vi "Node - Get Imported Ch Data.vi"(8 "error in (no error)":errorcluster) -> (0 "error out":errorcluster)   [LabVIEW 2016]
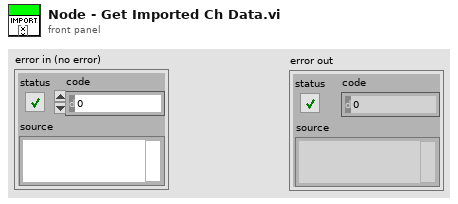
[diagram p1: front panel]
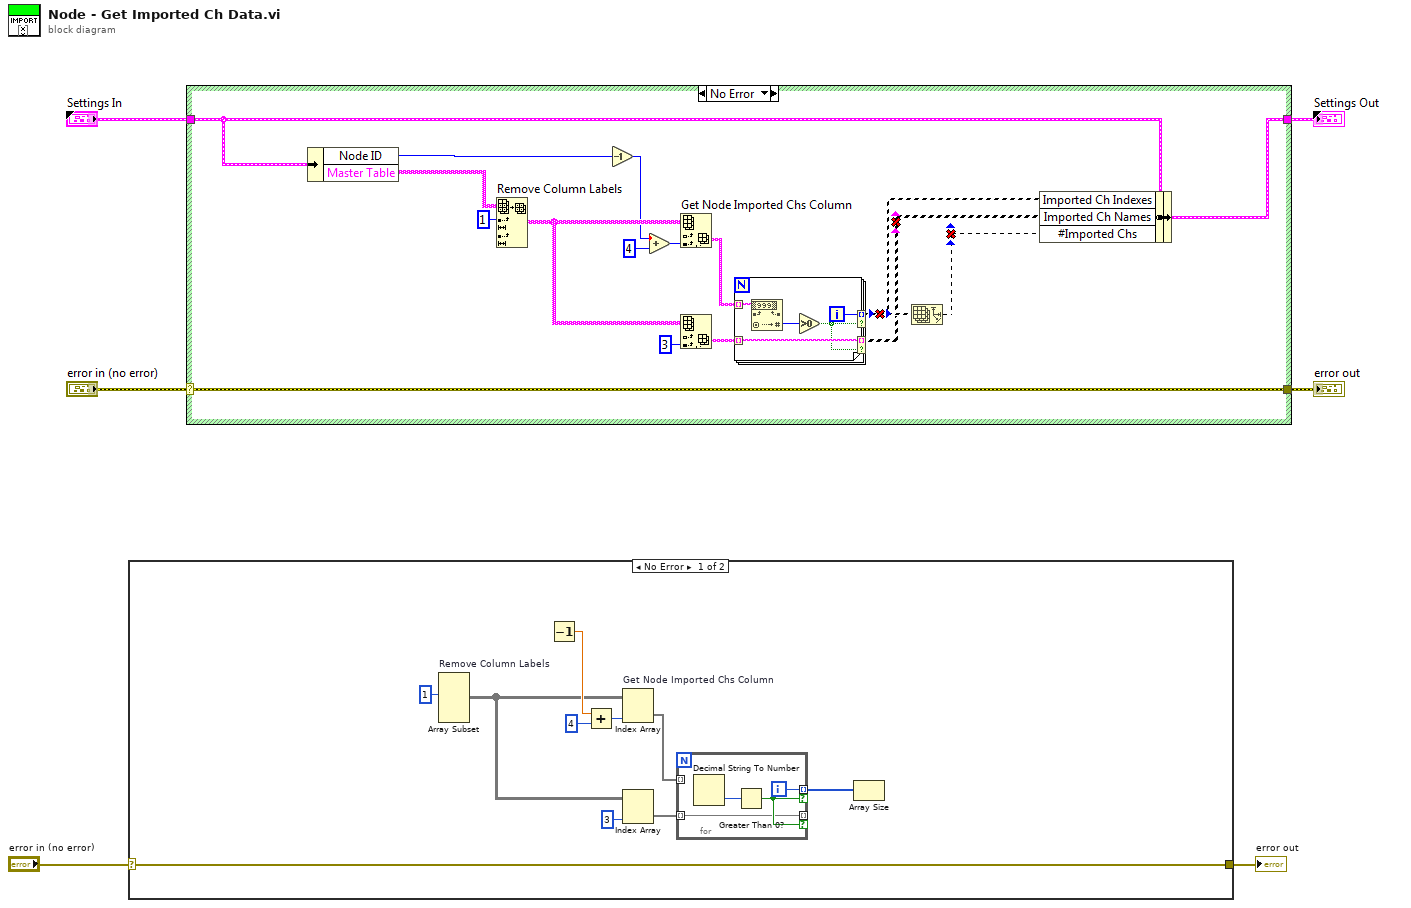
[diagram p0: block diagram]
diagram:
  n1 = case shown="No Error" "error in (no error)" {
    selector: "error in (no error)" -> [w6 w17]
    tunnel: [w6 w17] -> w1
    frame No Error {
      n2 = Array Subset "Remove Column Labels"(index (row)=1 ("index")) -> (w4:void[][])  [unwired: 4 in]
      n3 = Decrement() -> (x-1=w9:dbl)  [unwired: 1 in]
      n4 = Add(x=w9, y=4 ("index")) -> (x+y=w10:i32)
      n5 = Index Array "Get Node Imported Chs Column"(array=w4, index (col)=w10) -> (element=w8:void[])  [unwired: 1 in]
      n6 = Index Array(array=w4, index (col)=3 ("disabled index (col)")) -> (element=w3:void[])  [unwired: 1 in]
      n7 = for {
        tunnel: w8 -> [_] mode=indexing
        tunnel: [w15] -> w7 mode=indexing if=w14
        tunnel: [w13] -> _ mode=indexing if=w14
        tunnel: w3 -> [w13] mode=indexing
        i -> [w15]
        n8 = Decimal String To Number() -> (number=w16:i32)  [unwired: 3 in, 1 out]
        n9 = Greater Than 0?(x=w16) -> (x > 0?=w14:bool)
      }
      n10 = Array Size(array=w7) -> ()  [unwired: 1 out]
    }
    frame Error {
    }
  }
  "error out" <- w1
